vi "Single fast IV v1.0.vi"() -> ()   [LabVIEW 2023]
uses:
  RT fast data.ctl
  <vilib>/LabVIEW Targets/FPGA/cRIO/shared/nicrio_ModuleControls/nicrio_cRIO-9775_RecordDataRates4ChansRing.ctl
  <vilib>/Utility/file.llb/Write Delimited Spreadsheet (DBL).vi
  <resource>/objmgr/ni.dex.rc
panel:
  out "data file name":string="20230630-144537-Fast_IV.dat"
  in  "Sample Name":string
  out "Array":dbl[](array[numeric])
  in  "Tab Control":enum32{"cRIO", "IV parameters"}(tab)
  in  "cRIO IP":string="//172.22.11.2"
  in  "Data buffer size":i32=1000
  in  "Record Data Rate":T1=200 items=["20.000 MS/s (NI 9775)"=1, "10.00 MS/s (NI 9775)"=2, "6.667 MS/s (NI 9775)"=3, "5.000 MS/s (NI 9775)"=4, "2.500 MS/s (NI 9775)"=8, "1.667 MS/s (NI 9775)"=12, "1.250 MS/s (NI 9775)"=16, "1.000 MS/s (NI 9775)"=20, "833.333 KS/s (NI 9775)"=24, "714.286 KS/s (NI 9775)"=28, "625.000 KS/s (NI 9775)"=32, "555.556 KS/s (NI 9775)"=36, "500.000 KS/s (NI 9775)"=40, "454.545 KS/s (NI 9775)"=44, "416.667 KS/s (NI 9775)"=48, "384.615 KS/s (NI 9775)"=52, "357.143 KS/s (NI 9775)"=56, "333.333 KS/s (NI 9775)"=60, "312.500 KS/s (NI 9775)"=64, "294.118 KS/s (NI 9775)"=68, "277.778 KS/s (NI 9775)"=72, "263.158 KS/s (NI 9775)"=76, "250.000 KS/s (NI 9775)"=80, "238.095 KS/s (NI 9775)"=84, "227.273 KS/s (NI 9775)"=88, "217.391 KS/s (NI 9775)"=92, "208.333 KS/s (NI 9775)"=96, "200.000 KS/s (NI 9775)"=100, "192.308 KS/s (NI 9775)"=104, "185.185 KS/s (NI 9775)"=108, "178.571 KS/s (NI 9775)"=112, "172.414 KS/s (NI 9775)"=116, "166.667 KS/s (NI 9775)"=120, "161.290 KS/s (NI 9775)"=124, "156.250 KS/s (NI 9775)"=128, "151.515 KS/s (NI 9775)"=132, "147.059 KS/s (NI 9775)"=136, "142.857 KS/s (NI 9775)"=140, "138.889 KS/s (NI 9775)"=144, "135.135 KS/s (NI 9775)"=148, "131.579 KS/s (NI 9775)"=152, "128.205 KS/s (NI 9775)"=156, "125.000 KS/s (NI 9775)"=160, "121.951 KS/s (NI 9775)"=164, "119.048 KS/s (NI 9775)"=168, "116.279 KS/s (NI 9775)"=172, "113.636 KS/s (NI 9775)"=176, "111.111 KS/s (NI 9775)"=180, "108.696 KS/s (NI 9775)"=184, "106.383 KS/s (NI 9775)"=188, "104.167 KS/s (NI 9775)"=192, "102.041 KS/s (NI 9775)"=196, "100.000 KS/s (NI 9775)"=200, "50.000 KS/s (NI 9775)"=400, "33.333 KS/s (NI 9775)"=600, "25.000 KS/s (NI 9775)"=800, "20.000 KS/s (NI 9775)"=1000, "16.667 KS/s (NI 9775)"=1200, "14.286 KS/s (NI 9775)"=1400, "12.500 KS/s (NI 9775)"=1600, "11.111 KS/s (NI 9775)"=1800, "10.000 KS/s (NI 9775)"=2000, "9.091 KS/s (NI 9775)"=2200, "8.333 KS/s (NI 9775)"=2400, "7.692 KS/s (NI 9775)"=2600, "7.143 KS/s (NI 9775)"=2800, "6.667 KS/s (NI 9775)"=3000, "6.250 KS/s (NI 9775)"=3200, "5.882 KS/s (NI 9775)"=3400, "5.556 KS/s (NI 9775)"=3600, "5.000 KS/s (NI 9775)"=4000, "4.762 KS/s (NI 9775)"=4200, "4.545 KS/s (NI 9775)"=4400, "4.348 KS/s (NI 9775)"=4600, "4.167 KS/s (NI 9775)"=4800, "4.000 KS/s (NI 9775)"=5000, "3.846 KS/s (NI 9775)"=5200, "3.571 KS/s (NI 9775)"=5600, "3.333 KS/s (NI 9775)"=6000, "3.125 KS/s (NI 9775)"=6400, "2.941 KS/s (NI 9775)"=6800, "2.778 KS/s (NI 9775)"=7200, "2.632 KS/s (NI 9775)"=7600, "2.500 KS/s (NI 9775)"=8000, "2.381 KS/s (NI 9775)"=8400, "2.273 KS/s (NI 9775)"=8800, "2.174 KS/s (NI 9775)"=9200, "2.083 KS/s (NI 9775)"=9600, "2.000 KS/s (NI 9775)"=10000, "1.923 KS/s (NI 9775)"=10400, "1.852 KS/s (NI 9775)"=10800, "1.786 KS/s (NI 9775)"=11200, "1.724 KS/s (NI 9775)"=11600, "1.667 KS/s (NI 9775)"=12000, "1.613 KS/s (NI 9775)"=12400, "1.563 KS/s (NI 9775)"=12800, "1.515 KS/s (NI 9775)"=13200, "1.471 KS/s (NI 9775)"=13600, "1.429 KS/s (NI 9775)"=14000, "1.389 KS/s (NI 9775)"=14400, "1.351 KS/s (NI 9775)"=14800, "1.316 KS/s (NI 9775)"=15200, "1.282 KS/s (NI 9775)"=15600, "1.250 KS/s (NI 9775)"=16000, "1.220 KS/s (NI 9775)"=16400, "1.190 KS/s (NI 9775)"=16800, "1.163 KS/s (NI 9775)"=17200, "1.136 KS/s (NI 9775)"=17600, "1.111 KS/s (NI 9775)"=18000, "1.087 KS/s (NI 9775)"=18400, "1.064 KS/s (NI 9775)"=18800, "1.042 KS/s (NI 9775)"=19200, "1.020 KS/s (NI 9775)"=19600, "1.000 KS/s (NI 9775)"=20000, "0.980 KS/s (NI 9775)"=20400, "0.962 KS/s (NI 9775)"=20800, "0.943 KS/s (NI 9775)"=21200, "0.926 KS/s (NI 9775)"=21600, "0.909 KS/s (NI 9775)"=22000, "0.893 KS/s (NI 9775)"=22400, "0.877 KS/s (NI 9775)"=22800, "0.862 KS/s (NI 9775)"=23200, "0.847 KS/s (NI 9775)"=23600, "0.833 KS/s (NI 9775)"=24000, "0.820 KS/s (NI 9775)"=24400, "0.806 KS/s (NI 9775)"=24800, "0.794 KS/s (NI 9775)"=25200, "0.781 KS/s (NI 9775)"=25600, "0.694 KS/s (NI 9775)"=28800, "0.625 KS/s (NI 9775)"=32000, "0.568 KS/s (NI 9775)"=35200, "0.521 KS/s (NI 9775)"=38400, "0.446 KS/s (NI 9775)"=44800, "0.391 KS/s (NI 9775)"=51200, "0.347 KS/s (NI 9775)"=57600, "0.313 KS/s (NI 9775)"=64000]
  in  "Gate wait time us":u32=150
  in  "Record Samples":u32=5000
  in  "Current Scale factor":dbl=10.0
  in  "Average num":i32=1
  in  "Voltage Scale factor":dbl=0.0001
  in  "Count ms half of T":u32=15
  in  "Wait before trigger us":u32=10100
  out "IV parameters":T2={"Records Num"=1, "AI Trigger Configuration"={"Trigger Slope"=enum."Positive", "Trigger Level"=0.10009765625, "Hystesis Value"=0.094970703125, "AI Channel"=0}, "Record PreTrigger Samples"=1, "Record Samples"=5000, "Ic Cut off or curve"=FALSE, "Gate wait time us"=150, "Record Data Rate"=200, "Count us half of T"=15, "Wait before trigger us"=10100, "Cutoff delay usec"=0} {"Record Data Rate" items=["20.000 MS/s (NI 9775)"=1, "10.00 MS/s (NI 9775)"=2, "6.667 MS/s (NI 9775)"=3, "5.000 MS/s (NI 9775)"=4, "2.500 MS/s (NI 9775)"=8, "1.667 MS/s (NI 9775)"=12, "1.250 MS/s (NI 9775)"=16, "1.000 MS/s (NI 9775)"=20, "833.333 KS/s (NI 9775)"=24, "714.286 KS/s (NI 9775)"=28, "625.000 KS/s (NI 9775)"=32, "555.556 KS/s (NI 9775)"=36, "500.000 KS/s (NI 9775)"=40, "454.545 KS/s (NI 9775)"=44, "416.667 KS/s (NI 9775)"=48, "384.615 KS/s (NI 9775)"=52, "357.143 KS/s (NI 9775)"=56, "333.333 KS/s (NI 9775)"=60, "312.500 KS/s (NI 9775)"=64, "294.118 KS/s (NI 9775)"=68, "277.778 KS/s (NI 9775)"=72, "263.158 KS/s (NI 9775)"=76, "250.000 KS/s (NI 9775)"=80, "238.095 KS/s (NI 9775)"=84, "227.273 KS/s (NI 9775)"=88, "217.391 KS/s (NI 9775)"=92, "208.333 KS/s (NI 9775)"=96, "200.000 KS/s (NI 9775)"=100, "192.308 KS/s (NI 9775)"=104, "185.185 KS/s (NI 9775)"=108, "178.571 KS/s (NI 9775)"=112, "172.414 KS/s (NI 9775)"=116, "166.667 KS/s (NI 9775)"=120, "161.290 KS/s (NI 9775)"=124, "156.250 KS/s (NI 9775)"=128, "151.515 KS/s (NI 9775)"=132, "147.059 KS/s (NI 9775)"=136, "142.857 KS/s (NI 9775)"=140, "138.889 KS/s (NI 9775)"=144, "135.135 KS/s (NI 9775)"=148, "131.579 KS/s (NI 9775)"=152, "128.205 KS/s (NI 9775)"=156, "125.000 KS/s (NI 9775)"=160, "121.951 KS/s (NI 9775)"=164, "119.048 KS/s (NI 9775)"=168, "116.279 KS/s (NI 9775)"=172, "113.636 KS/s (NI 9775)"=176, "111.111 KS/s (NI 9775)"=180, "108.696 KS/s (NI 9775)"=184, "106.383 KS/s (NI 9775)"=188, "104.167 KS/s (NI 9775)"=192, "102.041 KS/s (NI 9775)"=196, "100.000 KS/s (NI 9775)"=200, "50.000 KS/s (NI 9775)"=400, "33.333 KS/s (NI 9775)"=600, "25.000 KS/s (NI 9775)"=800, "20.000 KS/s (NI 9775)"=1000, "16.667 KS/s (NI 9775)"=1200, "14.286 KS/s (NI 9775)"=1400, "12.500 KS/s (NI 9775)"=1600, "11.111 KS/s (NI 9775)"=1800, "10.000 KS/s (NI 9775)"=2000, "9.091 KS/s (NI 9775)"=2200, "8.333 KS/s (NI 9775)"=2400, "7.692 KS/s (NI 9775)"=2600, "7.143 KS/s (NI 9775)"=2800, "6.667 KS/s (NI 9775)"=3000, "6.250 KS/s (NI 9775)"=3200, "5.882 KS/s (NI 9775)"=3400, "5.556 KS/s (NI 9775)"=3600, "5.000 KS/s (NI 9775)"=4000, "4.762 KS/s (NI 9775)"=4200, "4.545 KS/s (NI 9775)"=4400, "4.348 KS/s (NI 9775)"=4600, "4.167 KS/s (NI 9775)"=4800, "4.000 KS/s (NI 9775)"=5000, "3.846 KS/s (NI 9775)"=5200, "3.571 KS/s (NI 9775)"=5600, "3.333 KS/s (NI 9775)"=6000, "3.125 KS/s (NI 9775)"=6400, "2.941 KS/s (NI 9775)"=6800, "2.778 KS/s (NI 9775)"=7200, "2.632 KS/s (NI 9775)"=7600, "2.500 KS/s (NI 9775)"=8000, "2.381 KS/s (NI 9775)"=8400, "2.273 KS/s (NI 9775)"=8800, "2.174 KS/s (NI 9775)"=9200, "2.083 KS/s (NI 9775)"=9600, "2.000 KS/s (NI 9775)"=10000, "1.923 KS/s (NI 9775)"=10400, "1.852 KS/s (NI 9775)"=10800, "1.786 KS/s (NI 9775)"=11200, "1.724 KS/s (NI 9775)"=11600, "1.667 KS/s (NI 9775)"=12000, "1.613 KS/s (NI 9775)"=12400, "1.563 KS/s (NI 9775)"=12800, "1.515 KS/s (NI 9775)"=13200, "1.471 KS/s (NI 9775)"=13600, "1.429 KS/s (NI 9775)"=14000, "1.389 KS/s (NI 9775)"=14400, "1.351 KS/s (NI 9775)"=14800, "1.316 KS/s (NI 9775)"=15200, "1.282 KS/s (NI 9775)"=15600, "1.250 KS/s (NI 9775)"=16000, "1.220 KS/s (NI 9775)"=16400, "1.190 KS/s (NI 9775)"=16800, "1.163 KS/s (NI 9775)"=17200, "1.136 KS/s (NI 9775)"=17600, "1.111 KS/s (NI 9775)"=18000, "1.087 KS/s (NI 9775)"=18400, "1.064 KS/s (NI 9775)"=18800, "1.042 KS/s (NI 9775)"=19200, "1.020 KS/s (NI 9775)"=19600, "1.000 KS/s (NI 9775)"=20000, "0.980 KS/s (NI 9775)"=20400, "0.962 KS/s (NI 9775)"=20800, "0.943 KS/s (NI 9775)"=21200, "0.926 KS/s (NI 9775)"=21600, "0.909 KS/s (NI 9775)"=22000, "0.893 KS/s (NI 9775)"=22400, "0.877 KS/s (NI 9775)"=22800, "0.862 KS/s (NI 9775)"=23200, "0.847 KS/s (NI 9775)"=23600, "0.833 KS/s (NI 9775)"=24000, "0.820 KS/s (NI 9775)"=24400, "0.806 KS/s (NI 9775)"=24800, "0.794 KS/s (NI 9775)"=25200, "0.781 KS/s (NI 9775)"=25600, "0.694 KS/s (NI 9775)"=28800, "0.625 KS/s (NI 9775)"=32000, "0.568 KS/s (NI 9775)"=35200, "0.521 KS/s (NI 9775)"=38400, "0.446 KS/s (NI 9775)"=44800, "0.391 KS/s (NI 9775)"=51200, "0.347 KS/s (NI 9775)"=57600, "0.313 KS/s (NI 9775)"=64000]}
  in  "Contour plot folder":path=path "C:/Users/gyue/Desktop/20230627 J_02"
  out "IV curve":cluster{"Y":dbl[], "Y":dbl[]}[](graph)
  out "error out":errorcluster
  # "Voltage x factor=uA"
  # "Voltage x factor=actual Volt"
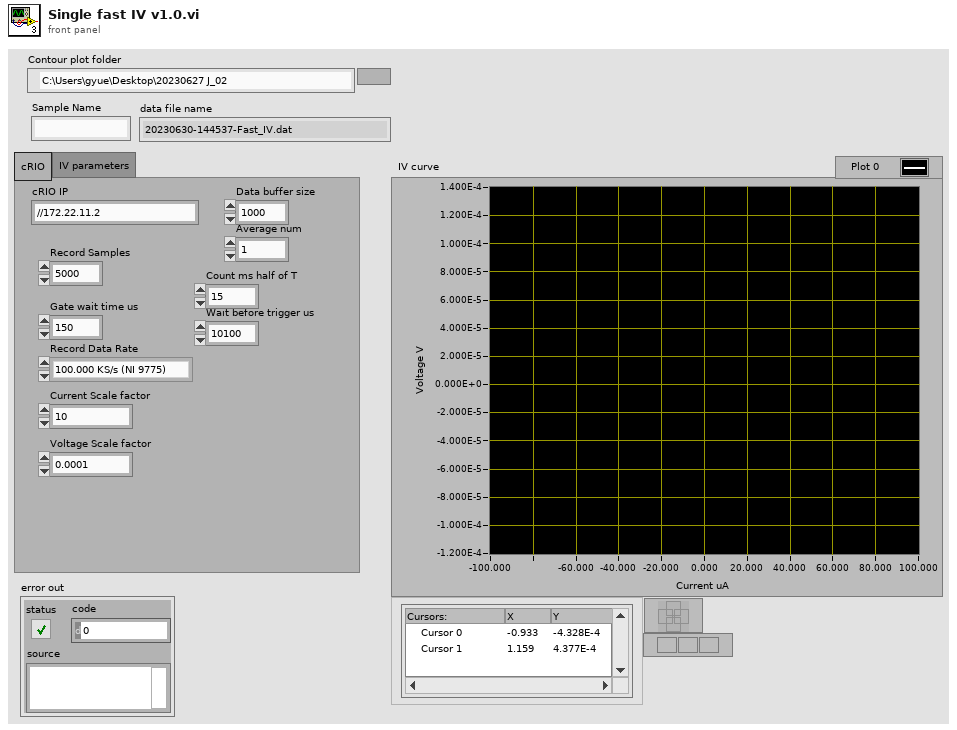
[diagram p1: front panel]
types:
  T1 = typedef "nicrio_cRIO-9775_RecordDataRates4ChansRing.ctl" = u16
  T2 = typedef "RT fast data.ctl" = cluster{"Records Num":i32, "AI Trigger Configuration":cluster{"Trigger Slope":enum8{"Positive", "Negative"}, "Trigger Level":fxp<+/-,17,5>, "Hystesis Value":fxp<+,16,4>, "AI Channel":u8}, "Record PreTrigger Samples":u32, "Record Samples":u32, "Ic Cut off or curve":bool, "Gate wait time us":u32, "Record Data Rate":T1, "Count us half of T":u32, "Wait before trigger us":u32, "Cutoff delay usec":u32}
  T3 = cluster{"Trigger Slope":enum8{"Positive", "Negative"}, "Trigger Level":fxp<+/-,17,5>, "Hystesis Value":fxp<+,16,4>, "AI Channel":u8}
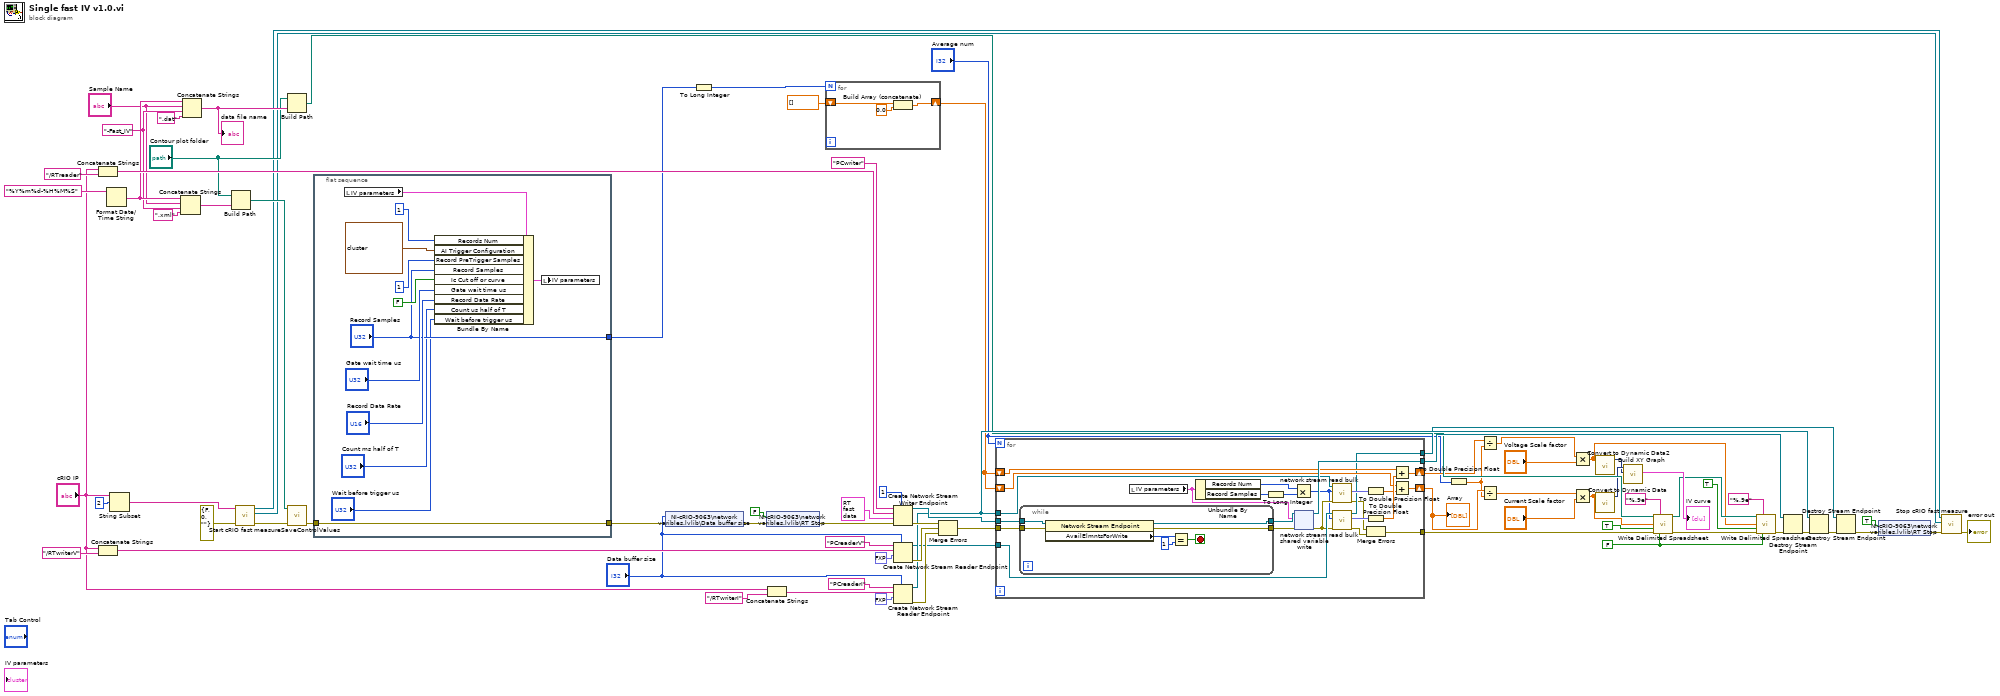
[diagram p0: block diagram]
diagram:
  w23 = FALSE ("transpose? (no:F)")
  w38 = "-Fast_IV"
  n1 = Concatenate Strings("cRIO IP", "/RTreader" ("string")) -> (w74:string)
  n2 = Concatenate Strings("cRIO IP", "/RTwriterV" ("string")) -> (w68:string)
  n3 = Format Date/Time String(time format string (%c)="%Y%m%d-%H%M%S") -> (date/time string=w39:string)  [unwired: 2 in]
  n4 = String Subset(string="cRIO IP", offset (0)=2) -> (substring=w1:string)  [unwired: 1 in]
  n5 = Concatenate Strings(w39, "Sample Name", w38, ".xml" ("string")) -> (w49:string)
  n6 = Concatenate Strings(w39, "Sample Name", w38, ".dat" ("string")) -> (w46:string)
  "data file name" <- w46
  n7 = Build Path(base path="Contour plot folder", name or relative path=w49) -> (appended path=w47:path)
  n8 = call "Start cRIO fast measure.vi"("error in (no error)"=errorcluster {"status"=FALSE, "code"=0, "source"=""} ("error in"), "machine IP"=w1) -> ("error out"=w8:errorcluster, "vi reference"=w6:refnum<vi>, "application reference"=w7:refnum<vi>)  [unwired: 7 in]
  n9 = Build Path(base path="Contour plot folder", name or relative path=w46) -> (appended path=w44:path)
  n10 = call "SaveControlValues.vi"("XML File Path"=w47, "error in (no error)"=w8) -> ("error out"=w40:errorcluster)  [unwired: 8 in]
  n11 = flat-sequence {
    tunnel: w40 -> [w90]
    tunnel: [w90] -> w43
    tunnel: ["Record Samples"] -> w42
    frame #0 {
      n12 = local read "IV parameters"() -> (w89:T2)
      n13 = Bundle By Name(cluster=w89, "Records Num"=1, "AI Trigger Configuration"=T3 {"Trigger Slope"=enum."Positive", "Trigger Level"=0.10009765625, "Hystesis Value"=0.094970703125, "AI Channel"=0}, "Record PreTrigger Samples"=u32 1, "Record Samples"="Record Samples", "Ic Cut off or curve"=FALSE, "Gate wait time us"="Gate wait time us", "Record Data Rate"="Record Data Rate", "Count us half of T"="Count ms half of T", "Wait before trigger us"="Wait before trigger us") -> (w83:T2)
      n14 = local write "IV parameters"(w83) -> ()
    }
  }
  n15 = shared-variable "NI-cRIO-9063\\network varibles.lvlib\\Data buffer size"("Data buffer size", error in=w43) -> (error out=w59:errorcluster)
  n16 = To Long Integer(number=w42) -> (32bit integer=w12:i32)
  n17 = shared-variable "NI-cRIO-9063\\network varibles.lvlib\\RT Stop"(FALSE ("RT Stop"), error in=w59) -> (error out=w66:errorcluster)
  n18 = Concatenate Strings("cRIO IP", "/RTwriterI" ("string")) -> (w61:string)
  n19 = for {
    N: w12 -> [_]
    shift-right: [w92] -> w15
    shift-left: dbl[] [] -> [w93]
    n20 = Build Array (concatenate)(w93, 0.0 ("new element/subarray")) -> (w92:dbl[])
  }
  n21 = Create Network Stream Writer Endpoint(7:1 ("writer buffer size"), 8:w66, 9:T2 {"Records Num"=0, "AI Trigger Configuration"={"Trigger Slope"=enum."Positive", "Trigger Level"=0.0, "Hystesis Value"=0.0, "AI Channel"=0}, "Record PreTrigger Samples"=0, "Record Samples"=0, "Ic Cut off or curve"=FALSE, "Gate wait time us"=0, "Record Data Rate"=1, "Count us half of T"=15, "Wait before trigger us"=10100, "Cutoff delay usec"=0} ("Parameters 4"), 10:w74, 11:"PCwriter" ("writer name")) -> (0:w72:errorcluster, 3:w71:refnum<k21>)  [unwired: 2 in]
  n22 = Create Network Stream Reader Endpoint(7:"Data buffer size", 9:fxp<+/-,17,5> 0.0, 10:w68, 11:"PCreaderV" ("reader name")) -> (0:w65:errorcluster, 3:w54:refnum<k21>)  [unwired: 3 in]
  n23 = Create Network Stream Reader Endpoint(7:"Data buffer size", 9:fxp<+/-,17,5> 0.0, 10:w61, 11:"PCreaderI" ("reader name")) -> (0:w58:errorcluster, 3:w56:refnum<k21>)  [unwired: 3 in]
  n24 = Merge Errors(w72, w65, w58) -> (w11:errorcluster)
  n25 = for {
    N: "Average num" -> [_]
    tunnel: w56 -> [w102]
    tunnel: w71 -> [w118]
    tunnel: [w116] -> w55
    tunnel: w54 -> [w101]
    tunnel: [w96] -> w53
    tunnel: w11 -> [w117]
    tunnel: [w109] -> w30
    shift-right: [w106] -> w24
    shift-left: w15 -> [w108]
    shift-right: [w104] -> w25
    shift-left: w15 -> [w103]
    n26 = while {
      tunnel: w118 -> [w125]
      tunnel: w117 -> [w124]
      tunnel: [w120] -> w115
      tunnel: [w119] -> w114
      stop <- w121 stop-if-true
      n27 = property class="Network Stream Endpoint"(reference=w125, error in=w124) -> (reference out=w120:refnum<k21>, error out=w119:errorcluster, "AvailElmntsForWrite"=w123:i32)
      n28 = Equal?(x=w123, y=1) -> (x = y?=w121:bool)
    }
    n29 = local read "IV parameters"() -> (w113:T2)
    n30 = Unbundle By Name(w113) -> ("Records Num"=w112:i32, "Record Samples"=w111:u32)
    n31 = To Long Integer(number=w111) -> (32bit integer=w110:i32)
    n32 = Multiply(x=w112, y=w110) -> (x*y=w99:i32)
    n33 = shared-variable-write(w115, w114, w113) -> (w116:refnum<k21>, w100:errorcluster)  [unwired: 1 in, 1 out]
    n34 = call "network stream read bulk.vi"("endpoint in"=w102, "Data num"=w99, "error in (no error)"=w100) -> ("Data"=w98:fxp<+/-,17,5>[], "error out"=w95:errorcluster)  [unwired: 5 in, 1 out]
    n35 = call "network stream read bulk.vi"("endpoint in"=w101, "Data num"=w99, "error in (no error)"=w100) -> ("endpoint out"=w96:refnum<k21>, "Data"=w97:fxp<+/-,17,5>[], "error out"=w94:errorcluster)  [unwired: 5 in]
    n36 = To Double Precision Float(number=w98) -> (double precision float=w105:dbl[])
    n37 = To Double Precision Float(number=w97) -> (double precision float=w107:dbl[])
    n38 = Merge Errors(w95, w94) -> (w109:errorcluster)
    n39 = Add(x=w108, y=w107) -> (x+y=w106:dbl[])
    n40 = Add(x=w103, y=w105) -> (x+y=w104:dbl[])
  }
  "Array" <- w25
  n41 = To Double Precision Float(number="Average num") -> (double precision float=w22:dbl)
  n42 = Divide(x=w24, y=w22) -> (x/y=w19:dbl[])
  n43 = Divide(x=w25, y=w22) -> (x/y=w20:dbl[])
  n44 = Multiply(x=w19, y="Voltage Scale factor") -> (x*y=w13:dbl[])
  n45 = Multiply(x=w20, y="Current Scale factor") -> (x*y=w14:dbl[])
  n46 = call "Convert to Dynamic Data2"("Array"=w13) -> ("Dynamic Data Type"=w33:dynamicdata)  [unwired: 3 in]
  n47 = call "Convert to Dynamic Data"("Array"=w14) -> ("Dynamic Data Type"=w34:dynamicdata)  [unwired: 3 in]
  n48 = call "Build XY Graph"("Y Input"=w33, "X Input"=w34) -> ("XY Graph"=→"IV curve":cluster{"X":dbl[], "Y":dbl[]}[])  [unwired: 8 in, 1 out]
  n49 = call-poly <vilib>:"Write Delimited Spreadsheet.vi"("file path (dialog if empty)"=w44, "format (%.3f)"="%.9e", "1D data"=w14, "append to file? (new file:F)"=TRUE, "error in (no error)"=w30, "transpose? (no:F)"=w23) -> ("new file path (Not A Path if cancelled)"=w26:path, "error out"=w27:errorcluster)  [unwired: 8 in]
  n50 = call-poly <vilib>:"Write Delimited Spreadsheet.vi"("file path (dialog if empty)"=w26, "format (%.3f)"="%.9e", "1D data"=w13, "append to file? (new file:F)"=TRUE, "error in (no error)"=w27, "transpose? (no:F)"=w23) -> ("error out"=w52:errorcluster)  [unwired: 8 in, 1 out]
  n51 = Destroy Stream Endpoint(8:w52, 11:w55) -> (0:w64:errorcluster)
  n52 = Destroy Stream Endpoint(8:w64, 11:w56) -> (0:w57:errorcluster)
  n53 = Destroy Stream Endpoint(8:w57, 11:w53) -> (0:w41:errorcluster)
  n54 = shared-variable "NI-cRIO-9063\\network varibles.lvlib\\RT Stop"(TRUE ("stop"), error in=w41) -> (error out=w5:errorcluster)
  n55 = call "Stop cRIO fast measure.vi"("error in (no error)"=w5, "VI reference"=w6, "application reference"=w7) -> ("error out"=→"error out":errorcluster)  [unwired: 8 in]
